vi "Make.vi"(8 "error in (no error)":errorcluster, 9 "Item Refnum":refnum<vi>, 10 "Target":refnum<vi>, 11 "Concrete Message Scripter":refnum<class "Concrete Message Scripter.lvclass">) -> (0 "error out":errorcluster, 3 "Concrete Message Scripter out":refnum<class "Concrete Message Scripter.lvclass">)   [LabVIEW 2020, in "Message Maker.lvlib" / "Concrete Message Scripter.lvclass"]
uses:
  Concrete Message Scripter.lvclass
  Concrete Message Scripter.lvclass/Concrete Message Scripter.ctl
  Message Scripter/Message Scripter.lvclass
  <vilib>/ErrorRing/Error Ring.xnode
  <vilib>/Utility/error.llb/Error Cluster From Error Code.vi
  Coupled Message Scripter/Coupled Message Scripter.lvclass
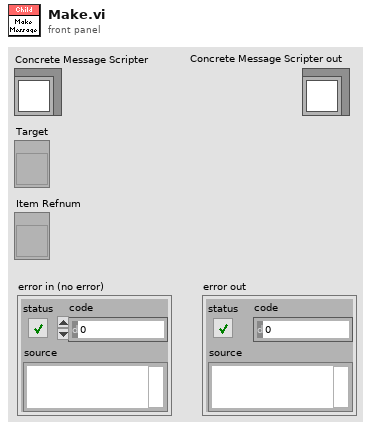
[diagram p1: front panel]
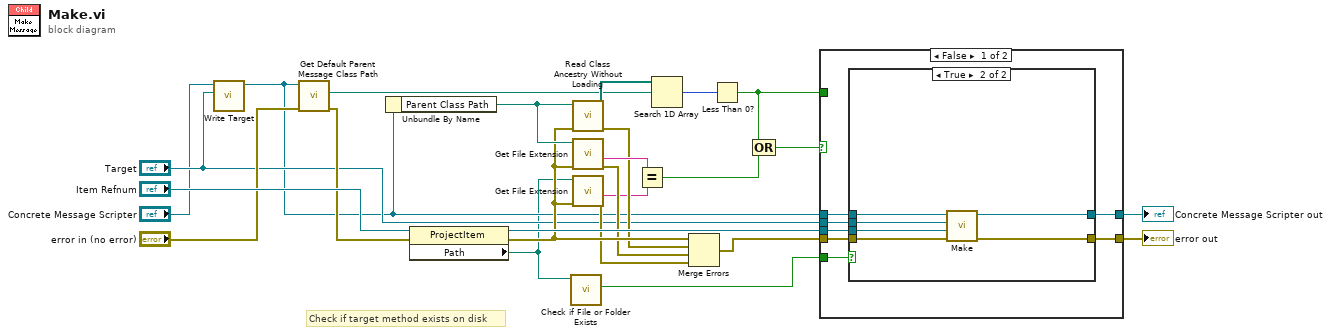
[diagram p0: block diagram]
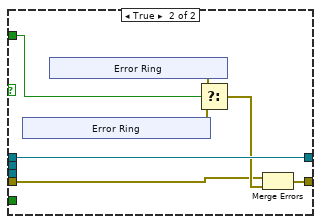
[diagram p3: hidden frame]
diagram:
  # "Check if target method exists on disk"
  n1 = call "Write Target.vi"("Target"="Target", "Message Scripter in"="Concrete Message Scripter") -> ("Message Scripter out"=w3:refnum<class "Concrete Message Scripter.lvclass">)  [unwired: 9 in]
  n2 = call "Get Default Parent Message Class Path.vi"("error in (no error)"="error in (no error)", "Message Scripter"=w3) -> ("error out"=w6:errorcluster, "Path String"=w7:path)  [unwired: 8 in]
  n3 = Unbundle By Name(w3) -> ("Parent Class Path"=w20:path)
  n4 = property class="ProjectItem"(reference="Item Refnum", error in=w6) -> (reference out=w22:refnum<vi>, error out=w19:errorcluster, "Path"=w2:path)
  n5 = call <vilib>:"Check if File or Folder Exists.vi"("path"=w2) -> ("file or folder exists?"=w1:bool)  [unwired: 8 in, 2 out]
  n6 = call <vilib>:"Read Class Ancestry Without Loading.vi"("error in (no error)"=w19, "LabVIEW Class Path"=w20) -> ("error out"=w16:errorcluster, "Class Ancestry"=w8:path[])  [unwired: 8 in]
  n7 = call <vilib>:"Get File Extension.vi"("error in (no error)"=w19, "file"=w20) -> ("error out"=w17:errorcluster, "filename without extension"=w21:string)  [unwired: 5 in, 3 out]
  n8 = call <vilib>:"Get File Extension.vi"("error in (no error)"=w19, "file"=w2) -> ("error out"=w18:errorcluster, "filename without extension"=w12:string)  [unwired: 5 in, 3 out]
  n9 = Equal?(x=w21, y=w12) -> (x = y?=w10:bool)
  n10 = Search 1D Array(1D array=w8, element=w7) -> (index of element=w9:i32)  [unwired: 1 in]
  n11 = Merge Errors(w19, w16, w17, w18) -> (w15:errorcluster)
  n12 = Less Than 0?(x=w9) -> (x < 0?=w11:bool)
  n13 = Compound Arithmetic op=OR(w11, w10) -> (w14:bool)
  n14 = case shown="False" w14 {
    tunnel: [w27 w42] -> w25
    tunnel: [w32 w47] -> w24
    tunnel: "Target" -> [w31 _]
    tunnel: w3 -> [w30 w47]
    tunnel: w22 -> [w29 _]
    tunnel: w15 -> [w28 w41]
    tunnel: w11 -> [_ w43]
    tunnel: w1 -> [w26 _]
    frame False {
      n15 = case shown="True" w26 {
        tunnel: [w34 w40] -> w32
        tunnel: w31 -> [_ w39]
        tunnel: w30 -> [w34 w38]
        tunnel: w29 -> [_ w37]
        tunnel: w28 -> [w33 w36]
        tunnel: [w33 w35] -> w27
        frame False {
        }
        frame True {
          n16 = call-parent "Make.vi"("error in (no error)"=w36, "Item Refnum"=w37, "Target"=w39, "Coupled Message Scripter"=w38) -> ("error out"=w35:errorcluster, "Coupled Message Scripter out"=w40:refnum<class "Concrete Message Scripter.lvclass">)  [unwired: 6 in]
        }
      }
    }
    frame True {
      n17 = xnode "Error Ring"() -> ("error out"=w46:errorcluster)
      n18 = xnode "Error Ring"() -> ("error out"=w45:errorcluster)
      n19 = Select(t=w45, s=w43, f=w46) -> (s? t:f=w44:errorcluster)
      n20 = Merge Errors(w41, w44) -> (w42:errorcluster)
    }
  }
  "error out" <- w25
  "Concrete Message Scripter out" <- w24
